vi "StopGlobal.vi"() -> ()   [LabVIEW 2025]
panel:
  out "inGame":bool
  in  "stop":bool
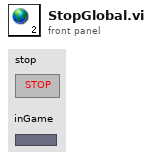
[diagram p1: front panel]
diagram:
